vi "DAC (A).vi"(8 "error in (no error)":errorcluster, 9 "voltage":dbl, 10 "channel":i32, 11 "Dac":refnum<k24>) -> (0 "error out":errorcluster)   [LabVIEW 2011]
doc: "Control the digital/analog converter manually (advanced version)."
uses:
  C:/Program Files/Metrohm Autolab/Autolab SDK 1.10/EcoChemie.Autolab.Sdk.dll
  EcoChemie.Autolab.Sdk.dll
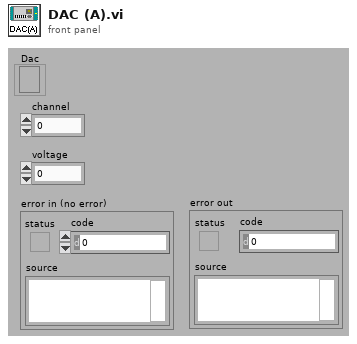
[diagram p1: front panel]
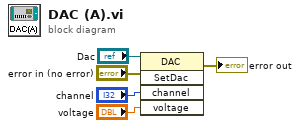
[diagram p0: block diagram]
diagram:
  n1 = invoke class="DAC" method="SetDac"(reference="Dac", error in="error in (no error)", "channel"="channel", "voltage"="voltage") -> (error out=→"error out":errorcluster)  [unwired: 1 in, 4 out]
